vi "Load Test.vi"(8 "error in":errorcluster, 11 "IED Test in":refnum<class "IED Test.lvclass">) -> (0 "error out":errorcluster, 2 "Test Result":T1=enum."Success", 3 "IED Test out":refnum<class "IED Test.lvclass">)   [LabVIEW 2018, in "IED Test Framework.lvlib" / "IED Test.lvclass"]
uses:
  IED Test.lvclass
  C:/Program Files (x86)/National Instruments/LabVIEW 2018/vi.lib/ActorFramework/Actor/Actor.lvclass
  Controls/Test Result.ctl
  <vilib>/ORNL/CSEISMIC DDS/CSEISMIC DDS Base/Data Types/Controls/DeviceClass Selector.ctl
  Load Actor/Load/Load.lvclass
  C:/Users/Administrator/Desktop/2018LabVIEW EMS/EMS Generic Actor/EMS Generic/EMS Generic.lvclass
  C:/Users/Administrator/Desktop/2018LabVIEW EMS/IED Actors/Device DDS Communications Framework/Device DDS Communications/Device DDS Communications.lvclass
  EMS Generic Actor/EMS Generic/EMS Generic.lvclass/EMS Generic.ctl
  <vilib>/ActorFramework/Message Enqueuer/Message Enqueuer.lvclass/Message Enqueuer.ctl
  <vilib>/ActorFramework/Message Enqueuer/Enqueue.vi
  <vilib>/ActorFramework/Stop Msg/Stop Msg.lvclass
  C:/Program Files (x86)/National Instruments/LabVIEW 2018/vi.lib/ActorFramework/Message/Message.lvclass
  <vilib>/ActorFramework/Message Priority Queue/Priority Enqueue.vi
  <vilib>/ORNL/CSEISMIC DDS/CSEISMIC DDS Base/CSEISMIC DDS.lvclass
  Device DDS Communications Framework/Device DDS Communications/Device DDS Communications.lvclass
  <vilib>/ActorFramework/Actor/Actor.lvclass
  EMS Generic Actor/EMS Generic/EMS Generic.lvclass
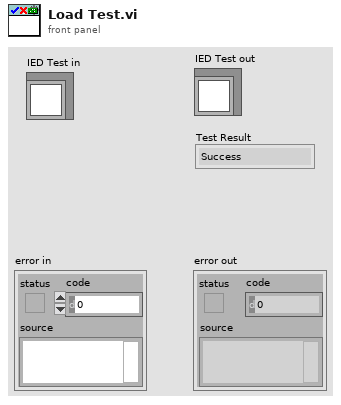
[diagram p1: front panel]
types:
  T1 = typedef "IED Test Framework.lvlib/IED Test.lvclass/Test Result.ctl" = enum16{"Invalid", "Success", "Failure", "Error", "Timeout"}
  T2 = typedef "CSEISMIC DDS.lvlib/CSEISMIC DDS.lvclass/DeviceClass Selector.ctl" = u16
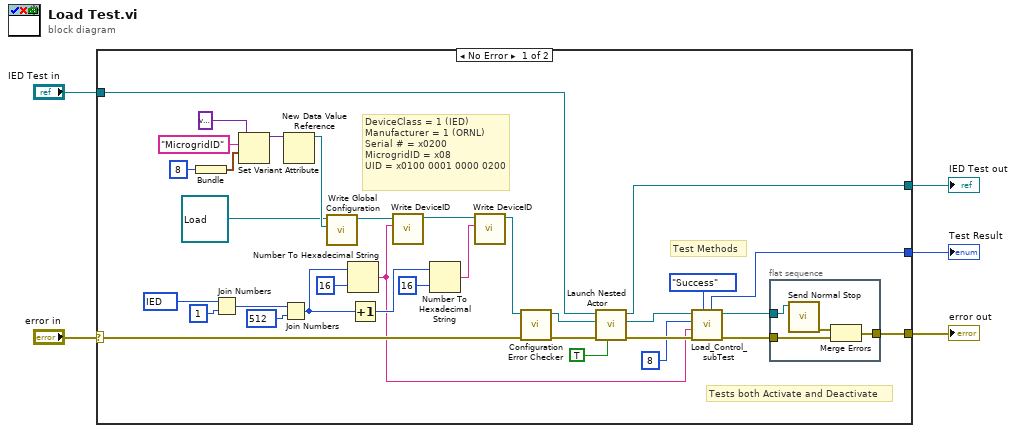
[diagram p0: block diagram]
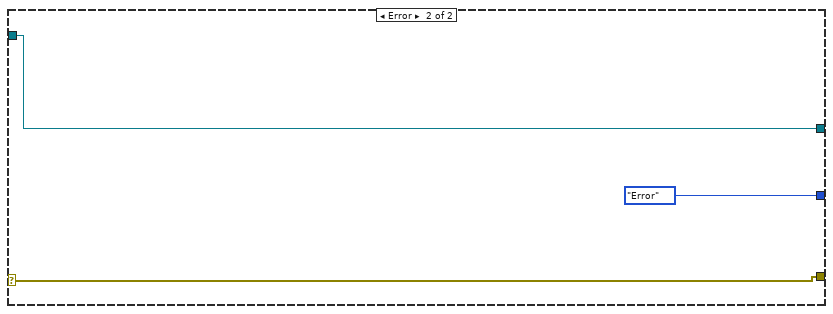
[diagram p2: hidden frame]
diagram:
  n1 = case shown="No Error" "error in" {
    selector: "error in" -> [w33 w46]
    tunnel: [w36 w46] -> w1
    tunnel: [w35 w45] -> w3
    tunnel: "IED Test in" -> [w37 w45]
    tunnel: [w12 Test_Result."Error" ("f")] -> w2
    frame No Error {
      w28 = T2 256 items=["Invalid"=0, "IED"=256, "DER"=512, "Relay"=768, "Meter"=1024, "Load"=1280, "Forecast"=1536, "Price"=1792, "Energy Storage"=513, "PV"=514, "Generator"=515, "Smart Relay"=769, "PCC"=770, "Smart Meter"=1025, "PMU"=1026, "HVAC"=1281] ("DeviceClass")
      # "DeviceClass = 1 (IED)\nManufacturer = 1 (ORNL)\nSerial # = x0200\nMicrogridID = x08\nUID = x0100 0001 0000 0200"
      # "Tests both Activate and Deactivate"
      # "Test Methods"
      n2 = Bundle("MicrogridID"=u8 8) -> (w6:cluster{"MicrogridID":u8})  [unwired: 1 in]
      n3 = Join Numbers(hi=w28, lo=u16 1 ("MicrogridID")) -> ((hi.lo)=w31:u32)
      n4 = Set Variant Attribute(Variant=variant ("variant"), name="MicrogridID", value=w6) -> (Variant out=w25:variant)  [unwired: 1 in, 2 out]
      n5 = Join Numbers(hi=w31, lo=u32 512 ("MicrogridID")) -> ((hi.lo)=w21:u64)
      n6 = New Data Value Reference(data value=w25) -> (data value reference=w24:refnum<data-value>)  [unwired: 1 in, 1 out]
      n7 = call "Write Global Configuration.vi"("Global Configuration"=w24, "EMS Generic in"=refnum<class "Load.lvclass"> refnum ("Load Actor.lvlib:Load.lvclass")) -> ("EMS Generic out"=w23:refnum<class "Load.lvclass">)  [unwired: 9 in]
      n8 = Number To Hexadecimal String(1:i16 16 ("width (-)"), 2:w21) -> (0:w10:string)
      n9 = Increment(x=w21) -> (x+1=w19:u64)
      n10 = call-dynamic "Write DeviceID.vi"("DeviceID"=w10, "Device DDS Communications in"=w23) -> ("Device DDS Communications out"=w29:refnum<class "Load.lvclass">)  [unwired: 9 in]
      n11 = Number To Hexadecimal String(1:i16 16 ("width (-)"), 2:w19) -> (0:w17:string)
      n12 = call-dynamic "Write DeviceID.vi"("DeviceID"=w17, "Device DDS Communications in"=w29) -> ("Device DDS Communications out"=w18:refnum<class "Load.lvclass">)  [unwired: 9 in]
      n13 = call "Configuration Error Checker.vi"("error in"=w33, "Device DDS Communications in"=w18) -> ("error out"=w38:errorcluster, "Device DDS Communications out"=w34:refnum<class "Load.lvclass">)  [unwired: 8 in]
      n14 = call <vilib>:"Launch Nested Actor.vi"("Open Actor Core front panel? (F)"=TRUE, "error in (no error)"=w38, "Nested Actor"=w34, "Caller Actor in"=w37) -> ("error out"=w15:errorcluster, "Nested Actor's Enqueuer"=w8:refnum<class "Message Enqueuer.lvclass">, "Caller Actor out"=w35:refnum<class "IED Test.lvclass">)  [unwired: 5 in]
      n15 = call "Load_Control_subTest.vi"("Test Result in"=Test_Result."Success", "error in"=w15, "DeviceID"=w10, "MicrogridID"=u8 8, "Message Enqueuer in"=w8) -> ("error out"=w14:errorcluster, "Message Enqueuer out"=w13:refnum<class "Message Enqueuer.lvclass">, "Test Result out"=w12:T1)  [unwired: 2 in, 2 out]
      n16 = flat-sequence {
        tunnel: w13 -> [w43]
        tunnel: [w41] -> w36
        tunnel: w14 -> [w40]
        frame #0 {
          n17 = call <vilib>:"Send Normal Stop.vi"("Message Enqueuer"=w43) -> ("error out"=w42:errorcluster)  [unwired: 10 in]
          n18 = Merge Errors(w42, w40) -> (w41:errorcluster)
        }
      }
    }
    frame Error {
    }
  }
  "error out" <- w1
  "IED Test out" <- w3
  "Test Result" <- w2
